vi "Kalman Filter CV Model (SubVI).vi"(0 "x":dbl, 5 "y":dbl, 7 "x-velocity":dbl, 9 "y-velocity":dbl, 11 "Error In":errorcluster) -> (4 "x corrected":dbl, 6 "y corrected":dbl, 8 "x-vel corrected":dbl, 10 "y-vel corrected":dbl, 15 "Error Out":errorcluster)   [LabVIEW 2017]
uses:
  <vilib>/addons/Control Design/_Stochastic Systems/Stochastic Systems.llb/Stochastic Systems SubVIs/cd_Stochastic State-Space Model.ctl
  <vilib>/addons/Control Design/_Stochastic Systems/Stochastic Systems.llb/Stochastic Systems SubVIs/cd_Second-Order Statistics Noise Model.ctl
  <vilib>/Simulation/Estimation/Implementation/NILVSim Discrete Kalman Filter.llb/SIM Disc KF Pred and Corr with Pred Gain with Checking Direct LV.vi
  <vilib>/Simulation/Implementation/XNodeFramework/SimXNode/SimX.xnode
  <vilib>/addons/Control Design/_Stochastic Systems/NI_CD_Stochastic Systems.lvlib
panel:
  # "Author: Steven Lee\nAim: This SubVI takes in the x, y, xdot, ydot from encoders and accelerometers and returns the corrected state estimate after they are processed using the Discrete Kalman Filter."
  # "from encoder"
  # "from encoder"
  # "from accelerometer"
  # "from accelerometer"
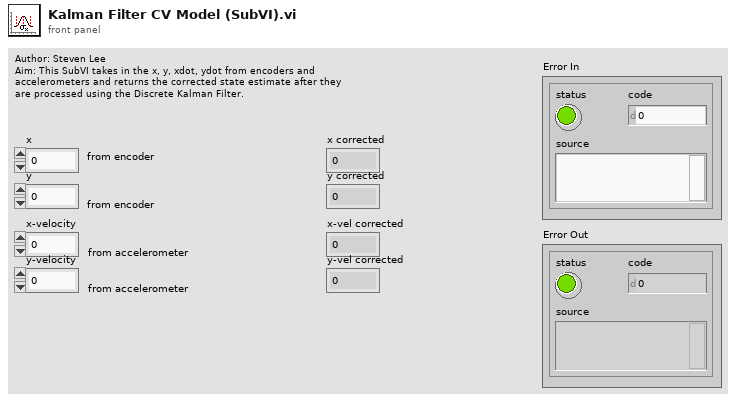
[diagram p1: front panel]
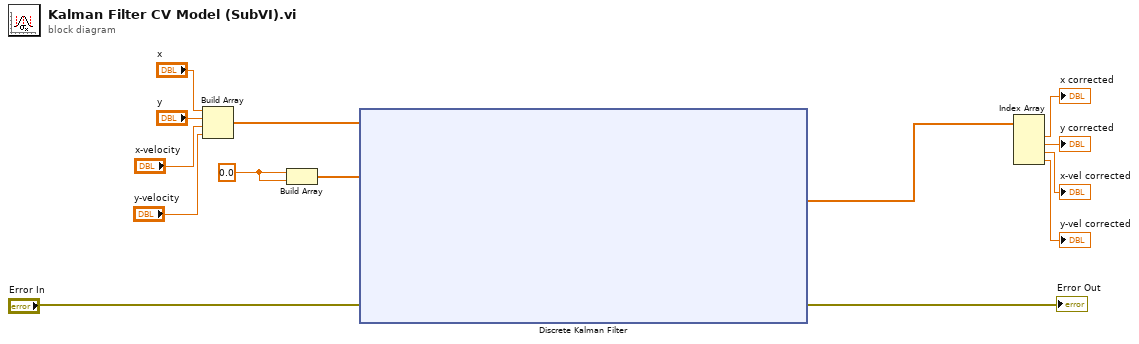
[diagram p0: block diagram]
diagram:
  w9 = 0.0 ("element")
  n1 = Build Array("x", "y", "x-velocity", "y-velocity") -> (w10:dbl[])
  n2 = Build Array(w9, w9) -> (w8:dbl[])
  n3 = xnode "Discrete Kalman Filter"("input u(k)"=w8, "Output y(k)"=w10, "error in (no error)"="Error In") -> ("Corrected State Estimate xhat(k|k)"=w5:dbl[], "error out"=→"Error Out":errorcluster)  [unwired: 1 in, 6 out]
  n4 = Index Array(array=w5) -> (element #1=→"x corrected":dbl, element #2=→"y corrected":dbl, element #3=→"x-vel corrected":dbl, element #4=→"y-vel corrected":dbl)  [unwired: 4 in]
